vi "VCM_Queue_Commands.vi"(1 "VCM Control":T1, 3 "VCM Queue":refnum<queue> caption="Mischer Levelmeter N") -> (0 "New Status":T1)   [LabVIEW 2019]
uses:
  Mischer/VCM-Control.ctl
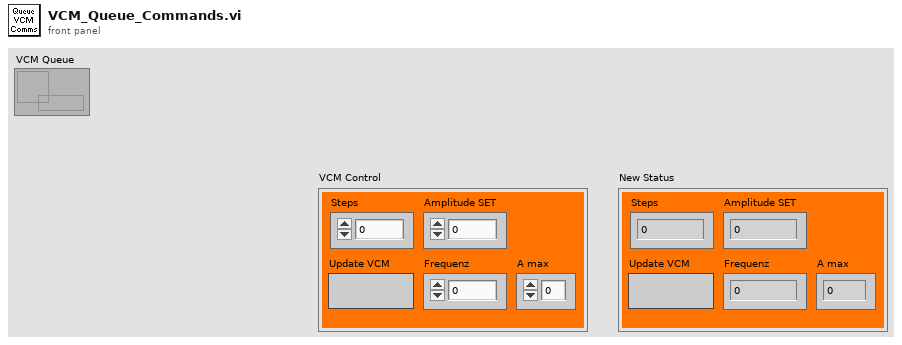
[diagram p1: front panel]
types:
  T1 = typedef "VCM-Control.ctl" = cluster{"Steps":dbl, "Amplitude SET":dbl, "Frequenz":dbl, "A max":dbl, "Update VCM":bool}
  T2 = cluster{"Steps":bool, "Amplitude SET":bool, "Frequenz":bool, "A max":bool, "Update VCM":bool}
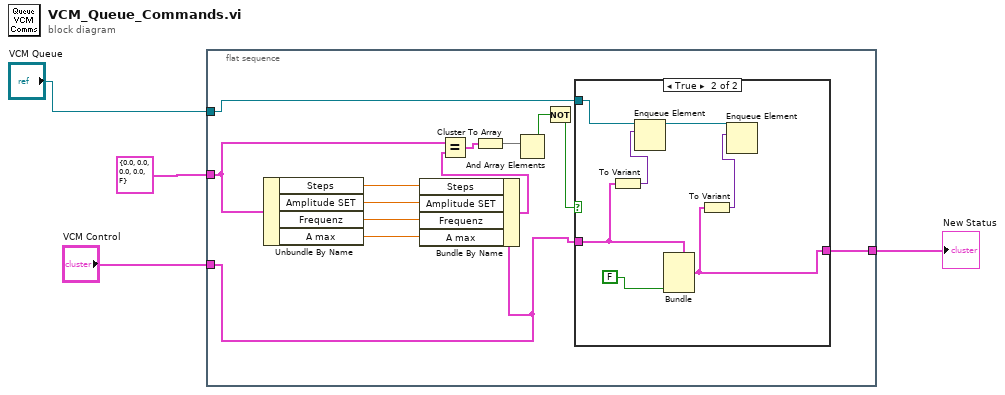
[diagram p0: block diagram]
diagram:
  n1 = flat-sequence {
    tunnel: "VCM Queue" -> [w7]
    tunnel: "VCM Control" -> [w6]
    tunnel: T1 {"Steps"=0.0, "Amplitude SET"=0.0, "Frequenz"=0.0, "A max"=0.0, "Update VCM"=FALSE} ("Last Status") -> [w17]
    tunnel: [w12] -> w1
    frame #0 {
      n2 = Unbundle By Name(w17) -> ("Steps"=w16:dbl, "Amplitude SET"=w15:dbl, "Frequenz"=w14:dbl, "A max"=w13:dbl)
      n3 = Bundle By Name(cluster=w6, "Steps"=w16, "Amplitude SET"=w15, "Frequenz"=w14, "A max"=w13) -> (w5:T1)
      n4 = Equal?(x=w17, y=w5) -> (x = y?=w11:T2)
      n5 = Cluster To Array(cluster=w11) -> (array=w10:bool[])
      n6 = And Array Elements(Boolean array=w10) -> (logical AND=w9:bool)
      n7 = Not(x=w9) -> (.not. x?=w8:bool)
      n8 = case shown="True" w8 {
        tunnel: w6 -> [w18 w22]
        tunnel: [w18 w20] -> w12
        tunnel: w7 -> [_ w25]
        frame False {
        }
        frame True {
          n9 = To Variant(anything=w22) -> (Variant=w23:variant)
          n10 = Enqueue Element(queue=w25, element=w23) -> (queue out=w24:refnum<queue>)  [unwired: 2 in, 2 out]
          n11 = Bundle(cluster=w22, "Update VCM"=FALSE) -> (w20:T1)  [unwired: 4 in]
          n12 = To Variant(anything=w20) -> (Variant=w21:variant)
          n13 = Enqueue Element(queue=w24, element=w21) -> ()  [unwired: 2 in, 3 out]
        }
      }
    }
  }
  "New Status" <- w1
